vi "Close.vi"(8 "error in (no error)":errorcluster, 9 "Responses in":T1[](array[typedef]) {"Command" items=["Constant Speed Tracking"=8, "Echo"=55, "Error"=255, "Home"=1, "Limit Active"=9, "Manual Move Tracking"=10, "Move Absolute"=20, "Move at Constant Speed"=22, "Move Relative"=21, "Renumber"=2, "Restore Settings"=36, "Stop"=23]}, 11 "VISA resource name":refnum<visa-resource-name>) -> (0 "error out":errorcluster, 1 "Responses out":T1[](array[typedef]) {"Command" items=["Constant Speed Tracking"=8, "Echo"=55, "Error"=255, "Home"=1, "Limit Active"=9, "Manual Move Tracking"=10, "Move Absolute"=20, "Move at Constant Speed"=22, "Move Relative"=21, "Renumber"=2, "Restore Settings"=36, "Stop"=23]})   [LabVIEW 2019, in "ZaberTSeries.lvlib"]
doc: "Terminates the software connection to the instrument. If you don't use Close, Labview won't complain but other applications won't be able to use the COM port."
uses:
  ZaberTSeries.lvlib
  Utility/Response.ctl
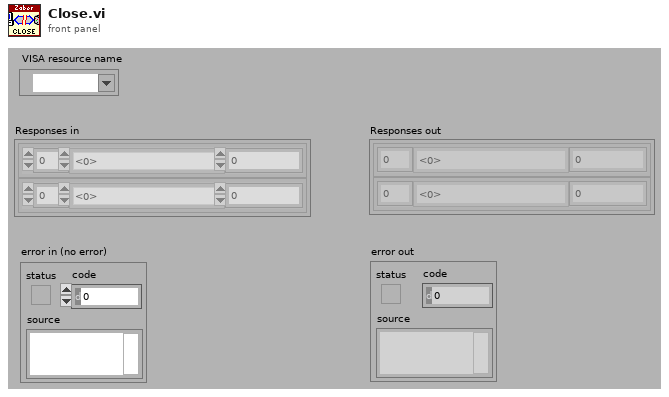
[diagram p1: front panel]
types:
  T1 = typedef "ZaberTSeries.lvlib/Response.ctl" = cluster{"Device Number":u8, "Command":u8, "Data":i32}
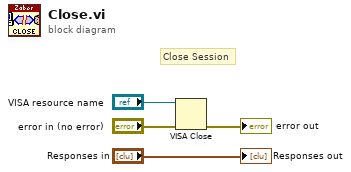
[diagram p0: block diagram]
diagram:
  # "Close Session"
  n1 = VISA Close(VISA resource name="VISA resource name", error in (no error)="error in (no error)") -> (error out=→"error out":errorcluster)
  "Responses out" <- "Responses in"
